vi "Get image delay.vi"(8 "error in (no error)":errorcluster, 11 "CCDCamera in":refnum<class "Real Camera.lvclass">) -> (0 "error out":errorcluster, 3 "CCDCamera out":refnum<class "Real Camera.lvclass">)   [LabVIEW 2018, in "Real Camera.lvclass"]
doc: "Get the delay of the start of an exposure from the start of a kinetic series.\n\nThis function should only be used in a kinetic series with two or more frames."
uses:
  Real Camera.lvclass
  C:/Users/Denis/Desktop/S4ACS/S4ACS/Simulated_CCD_Camera/Simulated Camera.lvclass
  Simulated_CCD_Camera/Simulated Camera.lvclass
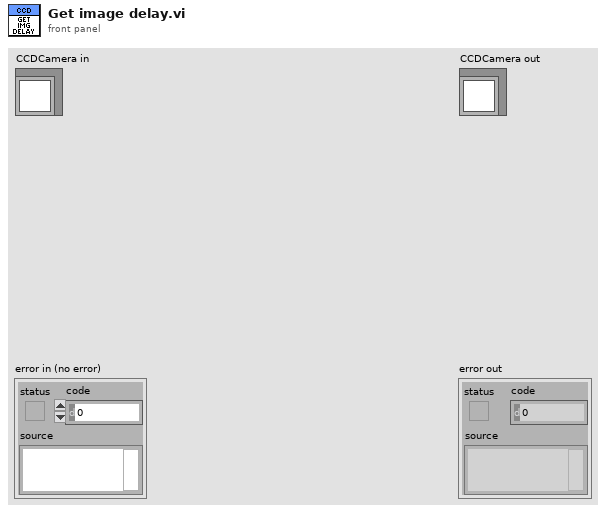
[diagram p1: front panel]
types:
  T1 = cluster{"CYCLES_DONE":u16, "LAST_IMAGE_NAME":string, "USED_DISK_SPACE":u16, "FRAMES_DONE":u16, "CCD_STATUS":string, "CURRENT_TEMPERATURE":i16, "TEMPERATURE_STATUS":string, "FRAME_EXPOSURE_TIME":sgl, "ERROR":bool, "SERIAL_NUMBER":u16, "ACQUIRING":bool, "IMAGE_INDEX":u32, "SEQS_DONE":u16, "ACS MODE":bool}
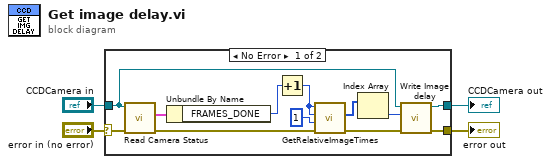
[diagram p0: block diagram]
diagram:
  n1 = case shown="No Error" "error in (no error)" {
    selector: "error in (no error)" -> [w10 w17]
    tunnel: "CCDCamera in" -> [w8 w18]
    tunnel: [w16 w18] -> w2
    tunnel: [w15 w17] -> w1
    frame No Error {
      n2 = call "Read Camera Status.vi"("error in (no error)"=w10, "CCDCamera in"=w8) -> ("error out"=w9:errorcluster, "Camera Status"=w7:T1)  [unwired: 7 in, 1 out]
      n3 = Unbundle By Name(w7) -> ("FRAMES_DONE"=w6:u16)
      n4 = Increment(x=w6) -> (x+1=w5:u16)
      n5 = call <userlib>:"GetRelativeImageTimes.vi"("error in (no error)"=w9, "size"=u32 1 ("first"), "last"=w5, "first"=w5) -> ("error out"=w12:errorcluster, "arr"=w13:u64[])  [unwired: 5 in, 1 out]
      n6 = Index Array(array=w13) -> (element=w11:u64)  [unwired: 1 in]
      n7 = call-dynamic "Write Image delay.vi"("error in (no error)"=w12, "Image delay"=w11, "Simulated_CCD_Camera in"=w8) -> ("error out"=w15:errorcluster, "Simulated_CCD_Camera out"=w16:refnum<class "Real Camera.lvclass">)  [unwired: 7 in]
    }
    frame Error {
    }
  }
  "error out" <- w1
  "CCDCamera out" <- w2
